vi "Inverse Kinematics.vi"(8 "Radii":T2 {"RB radius" format="%.2f"; "RF radius" format="%.2f"; "LB radius" format="%.2f"; "LF radius" format="%.2f"}, 11 "Target Velocity":dbl[](array[numeric]) format="%.2f") -> (0 "RB Pod Setpoint":cluster{"Velocity":dbl, "Theta":dbl}, 1 "RF Pod Setpoint":cluster{"Velocity":dbl, "Theta":dbl}, 2 "LB Pod Setpoint":cluster{"Velocity":dbl, "Theta":dbl}, 3 "LF Pod Setpoint":cluster{"Velocity":dbl, "Theta":dbl}, 5 "A x B":T1)   [LabVIEW 2020]
uses:
  <vilib>/Analysis/Matrix/Datatypes/RealMatrix.ctl
  <vilib>/Analysis/_algsub.llb/Real Vector Norm.vi
  <vilib>/Analysis/baseanly.llb/Real A x B.vi
  <vilib>/Analysis/Matrix/Numeric/Conversions/Array To Matrix - RA.vi
  <vilib>/Analysis/NI_AALPro.lvlib
  <vilib>/Analysis/Matrix/NI_Matrix.lvlib
  <vilib>/Analysis/NI_AALBase.lvlib
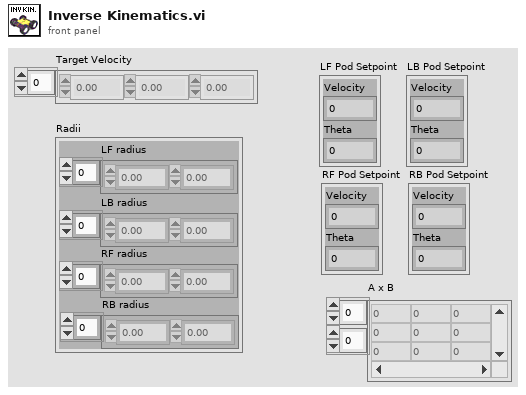
[diagram p1: front panel]
types:
  T1 = typedef "NI_Matrix.lvlib/RealMatrix.ctl" = dbl[][]
  T2 = cluster{"LF radius":dbl[], "LB radius":dbl[], "RF radius":dbl[], "RB radius":dbl[]}
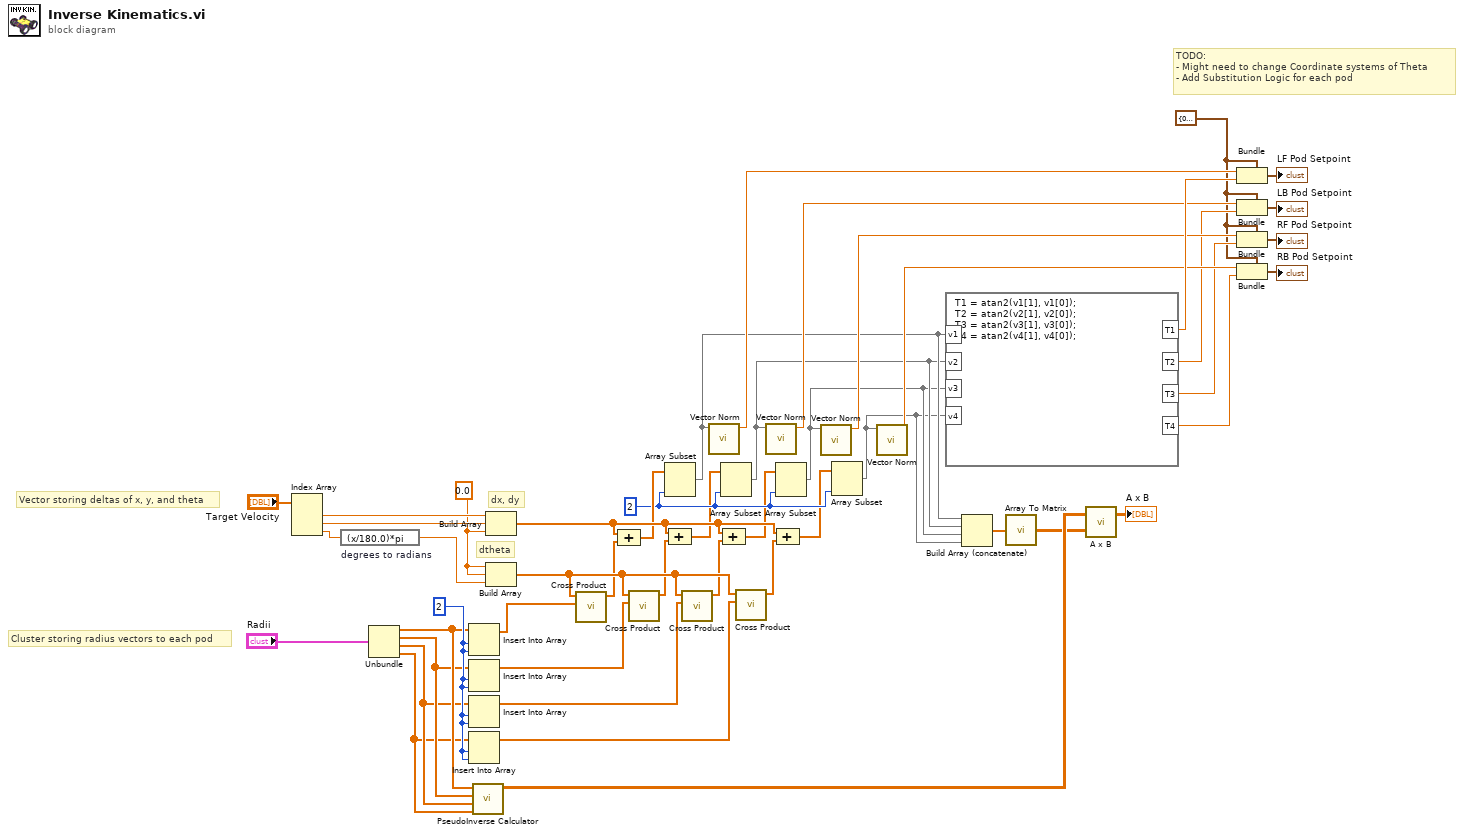
[diagram p0: block diagram]
diagram:
  w19 = 2 ("index")
  w24 = cluster{"Velocity":dbl, "Theta":dbl} {"Velocity"=0.0, "Theta"=0.0} ("Pod Setpoints")
  w36 = 2 ("length")
  w45 = 0.0 ("element")
  # "TODO: \n- Might need to change Coordinate systems of Theta\n- Add Substitution Logic for each pod"
  # "dtheta"
  # "dx, dy"
  # "Cluster storing radius vectors to each pod"
  # "Vector storing deltas of x, y, and theta"
  n1 = Index Array(array="Target Velocity") -> (element #1=w47:dbl, element #2=w46:dbl, element #3=w14:dbl)  [unwired: 3 in]
  n2 = expression code="(x/180.0)*pi" "degrees to radians"(w14) -> (w13:dbl)
  n3 = Unbundle("Radii") -> ("LF radius"=w12:dbl[], "LB radius"=w11:dbl[], "RF radius"=w10:dbl[], "RB radius"=w9:dbl[])
  n4 = Insert Into Array(array=w12, index=w19, new element=w19) -> (w18:dbl[])
  n5 = Insert Into Array(array=w11, index=w19, new element=w19) -> (w17:dbl[])
  n6 = Insert Into Array(array=w10, index=w19, new element=w19) -> (w16:dbl[])
  n7 = Insert Into Array(array=w9, index=w19, new element=w19) -> (w15:dbl[])
  n8 = call "PseudoInverse Calculator.vi"("R4"=w9, "R3"=w10, "R2"=w11, "R1"=w12) -> ("Pseudoinverse"=w3:T1)  [unwired: 7 in]
  n9 = Build Array(w47, w46, w45) -> (w38:dbl[])
  n10 = Build Array(w45, w45, w13) -> (w43:dbl[])
  n11 = call <vilib>:"Cross Product.vi"("B Vector"=w18, "A Vector"=w43) -> ("Cross Product"=w42:dbl[])  [unwired: 8 in, 1 out]
  n12 = Compound Arithmetic op=ADD(w38, w42) -> (w37:dbl[])
  n13 = call <vilib>:"Cross Product.vi"("B Vector"=w17, "A Vector"=w43) -> ("Cross Product"=w41:dbl[])  [unwired: 8 in, 1 out]
  n14 = Array Subset(array=w37, length=w36) -> (w8:dbl[])  [unwired: 1 in]
  n15 = Compound Arithmetic op=ADD(w38, w41) -> (w35:dbl[])
  n16 = call <vilib>:"Cross Product.vi"("B Vector"=w16, "A Vector"=w43) -> ("Cross Product"=w40:dbl[])  [unwired: 8 in, 1 out]
  n17 = call-poly <vilib>:"Vector Norm.vi"("Input Vector"=w8) -> ("norm"=w32:dbl)  [unwired: 9 in, 1 out]
  n18 = Array Subset(array=w35, length=w36) -> (w7:dbl[])  [unwired: 1 in]
  n19 = Compound Arithmetic op=ADD(w38, w40) -> (w34:dbl[])
  n20 = call <vilib>:"Cross Product.vi"("B Vector"=w15, "A Vector"=w43) -> ("Cross Product"=w39:dbl[])  [unwired: 8 in, 1 out]
  n21 = call-poly <vilib>:"Vector Norm.vi"("Input Vector"=w7) -> ("norm"=w30:dbl)  [unwired: 9 in, 1 out]
  n22 = Array Subset(array=w34, length=w36) -> (w6:dbl[])  [unwired: 1 in]
  n23 = Compound Arithmetic op=ADD(w38, w39) -> (w33:dbl[])
  n24 = call-poly <vilib>:"Vector Norm.vi"("Input Vector"=w6) -> ("norm"=w29:dbl)  [unwired: 9 in, 1 out]
  n25 = Array Subset(array=w33, length=w36) -> (w5:dbl[])  [unwired: 1 in]
  n26 = call-poly <vilib>:"Vector Norm.vi"("Input Vector"=w5) -> ("norm"=w28:dbl)  [unwired: 9 in, 1 out]
  n27 = formula code="T1 = atan2(v1[1], v1[0]);\nT2 = atan2(v2[1], v2[0]);\nT3 = atan2(v3[1], v3[0]);\nT4 = atan2(v4[1], v4[0]);"("v1"=w8, "v2"=w7, "v3"=w6, "v4"=w5) -> ("T1"=w31:dbl, "T2"=w27:dbl, "T3"=w26:dbl, "T4"=w25:dbl)
  n28 = Build Array (concatenate)(w8, w7, w6, w5) -> (w4:dbl[])
  n29 = call-poly <vilib>:"Array To Matrix.vi"("Real 1D Array"=w4) -> ("Real Matrix (Column Vector)"=w1:T1)
  n30 = call-poly <vilib>:"A x B.vi"("B"=w1, "A"=w3) -> ("A x B"=→"A x B":T1)  [unwired: 1 out]
  n31 = Bundle(cluster=w24, "Velocity"=w32, "Theta"=w31) -> (→"LF Pod Setpoint":cluster{"Velocity":dbl, "Theta":dbl})
  n32 = Bundle(cluster=w24, "Velocity"=w30, "Theta"=w27) -> (→"LB Pod Setpoint":cluster{"Velocity":dbl, "Theta":dbl})
  n33 = Bundle(cluster=w24, "Velocity"=w29, "Theta"=w26) -> (→"RF Pod Setpoint":cluster{"Velocity":dbl, "Theta":dbl})
  n34 = Bundle(cluster=w24, "Velocity"=w28, "Theta"=w25) -> (→"RB Pod Setpoint":cluster{"Velocity":dbl, "Theta":dbl})
